vi "StartCloudGrid.vi"(1 "error in (no error)":errorcluster) -> (0 "error out":errorcluster)   [LabVIEW 2014]
panel:
  in  "AutoItX3Lib.IAutoItX3":refnum<k7>
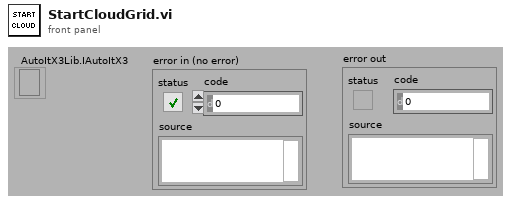
[diagram p1: front panel]
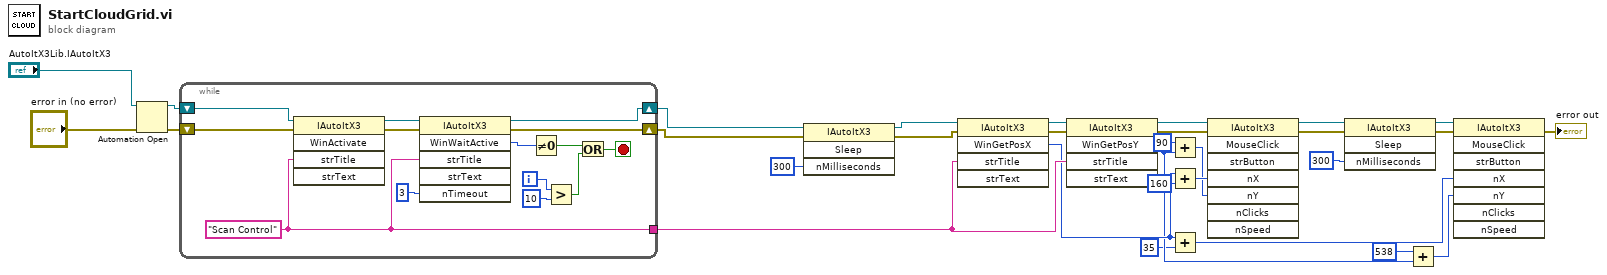
[diagram p0: block diagram]
diagram:
  n1 = Automation Open(error in (no error)="error in (no error)", Automation Refnum="AutoItX3Lib.IAutoItX3") -> (Automation Refnum=w25:refnum<k7>, error out=w26:errorcluster)  [unwired: 2 in]
  n2 = while {
    shift-right: [w43] -> w5
    shift-left: w26 -> [w42]
    shift-right: [w44] -> w4
    shift-left: w25 -> [w40]
    tunnel: [w31] -> w17
    i -> [w37]
    stop <- w33 stop-if-true
    w31 = "Scan Control" ("strTitle")
    n3 = invoke class="IAutoItX3" method="WinActivate"(reference=w40, error in=w42, "strTitle"=w31) -> (reference out=w39:refnum<k7>, error out=w41:errorcluster)  [unwired: 2 in, 3 out]
    n4 = invoke class="IAutoItX3" method="WinWaitActive"(reference=w39, error in=w41, "strTitle"=w31, "nTimeout"=3) -> (reference out=w44:refnum<k7>, error out=w43:errorcluster, "WinWaitActive"=w32:i32)  [unwired: 2 in, 3 out]
    n5 = Not Equal To 0?(x=w32) -> (x != 0?=w35:bool)
    n6 = Greater?(x=w37, y=10) -> (0:w34:bool)
    n7 = Or(x=w35, y=w34) -> (x .or. y?=w33:bool)
  }
  n8 = invoke class="IAutoItX3" method="Sleep"(reference=w4, error in=w5, "nMilliseconds"=300) -> (reference out=w3:refnum<k7>, error out=w2:errorcluster)  [unwired: 1 in, 2 out]
  n9 = invoke class="IAutoItX3" method="WinGetPosX"(reference=w3, error in=w2, "strTitle"=w17) -> (reference out=w29:refnum<k7>, error out=w28:errorcluster, "WinGetPosX"=w15:i32)  [unwired: 2 in, 2 out]
  n10 = invoke class="IAutoItX3" method="WinGetPosY"(reference=w29, error in=w28, "strTitle"=w17) -> (reference out=w24:refnum<k7>, error out=w22:errorcluster, "WinGetPosY"=w14:i32)  [unwired: 2 in, 2 out]
  n11 = Add(x=90, y=w14) -> (x+y=w10:i32)
  n12 = Add(x=w15, y=160) -> (x+y=w11:i32)
  n13 = Add(x=w15, y=35) -> (x+y=w12:i32)
  n14 = invoke class="IAutoItX3" method="MouseClick"(reference=w24, error in=w22, "nX"=w11, "nY"=w10) -> (reference out=w23:refnum<k7>, error out=w21:errorcluster)  [unwired: 4 in, 6 out]
  n15 = invoke class="IAutoItX3" method="Sleep"(reference=w23, error in=w21, "nMilliseconds"=300) -> (reference out=w20:refnum<k7>, error out=w19:errorcluster)  [unwired: 1 in, 2 out]
  n16 = Add(x=538, y=w14) -> (x+y=w13:i32)
  n17 = invoke class="IAutoItX3" method="MouseClick"(reference=w20, error in=w19, "nX"=w12, "nY"=w13) -> (error out=→"error out":errorcluster)  [unwired: 4 in, 7 out]
